vi "AKIP_set_voltage_current.vi"(8 "error in (no error)":errorcluster, 9 "Current":dbl, 10 "Voltage":dbl, 11 "VISA resource name (in)":refnum<visa-resource-name>="AKIP") -> (0 "error out":errorcluster, 3 "VISA resource name (out)":refnum<visa-resource-name>)   [LabVIEW 2017]
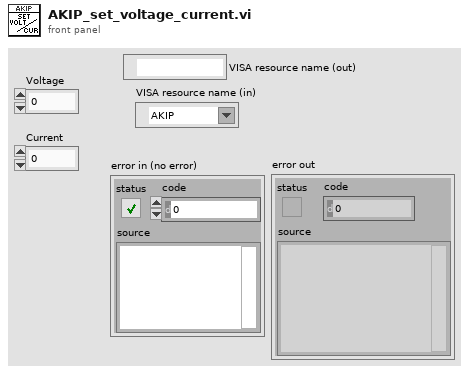
[diagram p1: front panel]
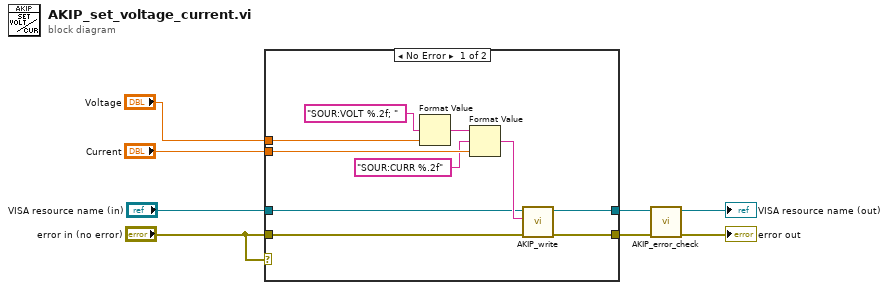
[diagram p0: block diagram]
diagram:
  n1 = case shown="No Error" "error in (no error)" {
    tunnel: "Voltage" -> [w17 _]
    tunnel: "Current" -> [w15 _]
    tunnel: "VISA resource name (in)" -> [w12 w20]
    tunnel: "error in (no error)" -> [w11 w19]
    tunnel: [w10 w19] -> w3
    tunnel: [w9 w20] -> w4
    frame No Error {
      n2 = Format Value(format string="SOUR:VOLT %.2f; " ("write buffer"), value (0)=w17) -> (output string=w18:string)  [unwired: 1 in]
      n3 = Format Value(string ("")=w18, format string="SOUR:CURR %.2f" ("write buffer"), value (0)=w15) -> (output string=w13:string)
      n4 = call "AKIP_write.vi"("error in (no error)"=w11, "write buffer"=w13, "VISA Refnum in"=w12) -> ("error out"=w10:errorcluster, "VISA Refnum out"=w9:refnum<visa-resource-name>)  [unwired: 7 in]
    }
    frame Error {
    }
  }
  n5 = call "AKIP_error_check.vi"("error in (no error)"=w3, "VISA Refnum in"=w4) -> ("error out"=→"error out":errorcluster, "VISA Refnum out"=→"VISA resource name (out)":refnum<visa-resource-name>)  [unwired: 8 in]
